vi "CBindInput.vi"(8 "error in (no error)":errorcluster, 10 "Authenticate Extra  Data":T1, 11 "WampScramAuthenticator in":refnum<class "WampScramAuthenticator.lvclass">) -> (0 "error out":errorcluster, 1 "CBindInput":string, 2 "Authenticate Extra Data":T1, 3 "WampScramAuthenticator out":refnum<class "WampScramAuthenticator.lvclass">)   [LabVIEW 2020, in "wamplv.lvlib" / "WampScramAuthenticator.lvclass"]
uses:
  WampScramAuthenticator.lvclass
  WampScramAuthenticator.lvclass/WampScramAuthenticator.ctl
  Utils/Utils.lvclass
  TypeDefs/Authenticate Extra data.ctl
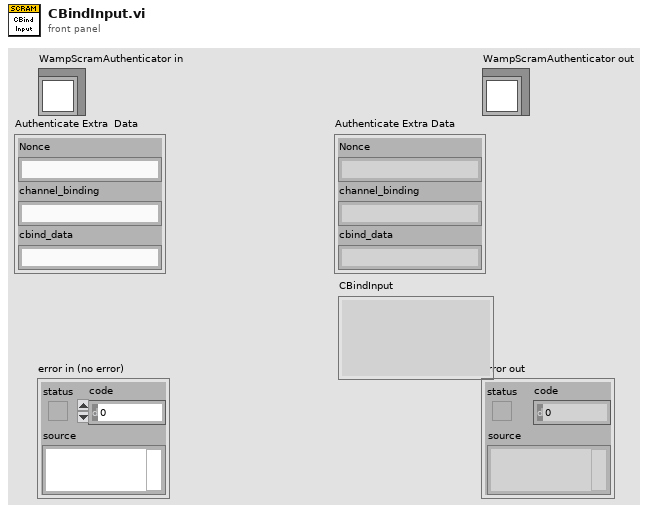
[diagram p1: front panel]
types:
  T1 = typedef "wamplv.lvlib/WampScramAuthenticator.lvclass/Authenticate Extra data.ctl" = cluster{"Nonce":string, "channel_binding":string, "cbind_data":string}
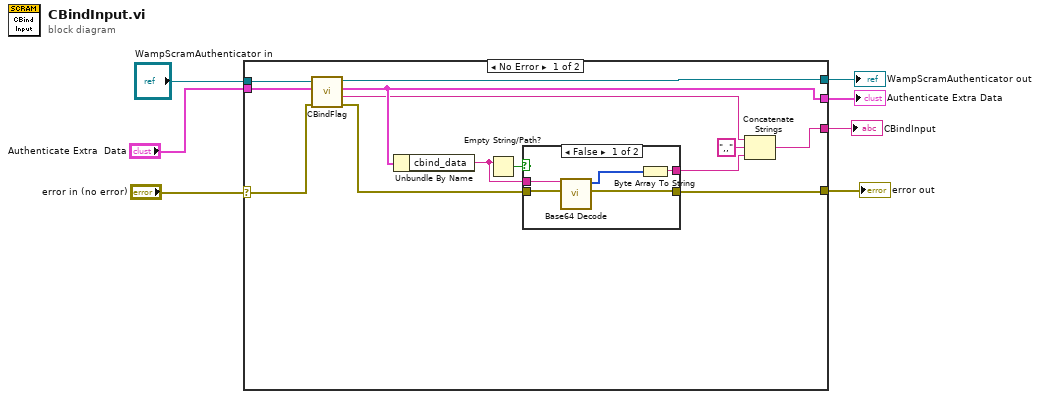
[diagram p0: block diagram]
diagram:
  n1 = case shown="No Error" "error in (no error)" {
    selector: "error in (no error)" -> [w17 w27]
    tunnel: "WampScramAuthenticator in" -> [w20 w29]
    tunnel: [w19 w29] -> w6
    tunnel: "Authenticate Extra  Data" -> [w18 w28]
    tunnel: [w16 w28] -> w3
    tunnel: [w8 _] -> w2
    tunnel: [w10 w27] -> w1
    frame No Error {
      n2 = call "CBindFlag.vi"("error in (no error)"=w17, "Authenticate Extra  Data"=w18, "WampScramAuthenticator in"=w20) -> ("error out"=w11:errorcluster, "CBindFlag"=w14:string, "Authenticate Extra  Data"=w16:T1, "WampScramAuthenticator out"=w19:refnum<class "WampScramAuthenticator.lvclass">)  [unwired: 5 in]
      n3 = Unbundle By Name(w16) -> ("cbind_data"=w12:string)
      n4 = Empty String/Path?(string/path=w12) -> (empty?=w13:bool)
      n5 = case shown="False" w13 {
        tunnel: w12 -> [w25 _]
        tunnel: w11 -> [w24 w26]
        tunnel: [w21 w26] -> w10
        tunnel: [w23 _] -> w9
        frame False {
          n6 = call "Base64 Decode.vi"("error in (no error)"=w24, "string in (base64-encoded)"=w25) -> ("error out"=w21:errorcluster, "Byte array"=w22:u8[])  [unwired: 8 in]
          n7 = Byte Array To String(unsigned byte array=w22) -> (string=w23:string)
        }
        frame True {
        }
      }
      n8 = Concatenate Strings(w14, ",," ("string"), w9) -> (w8:string)
    }
    frame Error {
    }
  }
  "error out" <- w1
  "WampScramAuthenticator out" <- w6
  "Authenticate Extra Data" <- w3
  "CBindInput" <- w2
